vi "Build Device Mask.vi"(0 "Device Idx (0-5)":u32, 7 "All Devices":bool) -> (4 "Socket Mask [U32]":u32=132 format="%06x", 8 "DUT Mask":bool[](array[boolean])=[TRUE, TRUE, TRUE, TRUE, TRUE, TRUE])   [LabVIEW 2017, in "Host SRL.lvlib"]
uses:
  Host SRL.lvlib
panel:
  # "Dev 01"
  # "Dev 02"
  # "Dev 03"
  # "Dev 04"
  # "Dev 05"
  # "Dev 06"
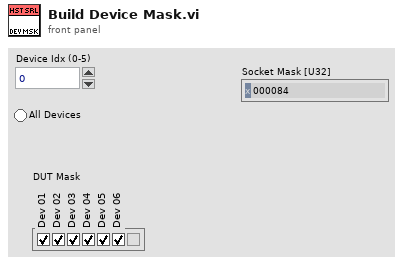
[diagram p1: front panel]
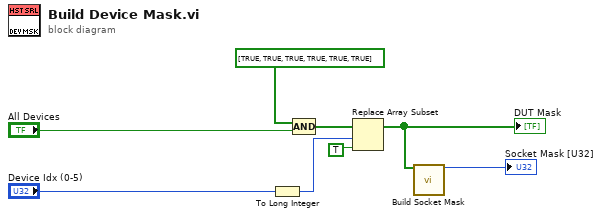
[diagram p0: block diagram]
diagram:
  n1 = To Long Integer(number="Device Idx (0-5)") -> (32bit integer=w4:i32)
  n2 = Compound Arithmetic op=AND(bool[] [TRUE, TRUE, TRUE, TRUE, TRUE, TRUE] ("DUT Mask"), "All Devices") -> (w7:bool[])
  n3 = Replace Array Subset(array=w7, new element=TRUE, index=w4) -> (w3:bool[])
  "DUT Mask" <- w3
  n4 = call "Build Socket Mask.vi"("Dev Mask (All)"=w3) -> ("Socket Mask [U32]"=→"Socket Mask [U32]":u32)  [unwired: 14 in]
